vi "Get Property.vi"(0 "Session Handle in":T1, 5 "resources":string, 7 "property":refnum<k21>, 11 "error in (no error)":errorcluster) -> (4 "Session Handle out":T1, 10 "property value":bool, 15 "error out":errorcluster)   [LabVIEW 2015, in "SLSC Switch.lvlib" / "SLSC Session.lvclass"]
uses:
  SLSC Session.lvclass
  Typedefs/Session Handle.ctl
  SLSC Session.lvclass/SLSC Session.ctl
  <vilib>/SLSC/Get Generic Property (Bool).vi
  <vilib>/SLSC/SLSC.lvlib
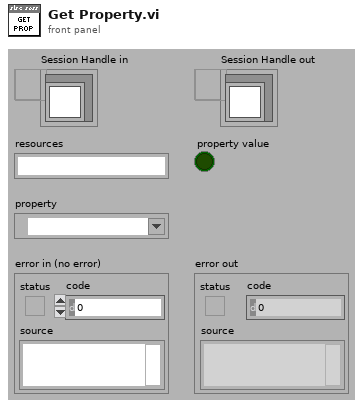
[diagram p1: front panel]
types:
  T1 = typedef "SLSC Switch.lvlib/SLSC Session.lvclass/Session Handle.ctl" = refnum<data-value>
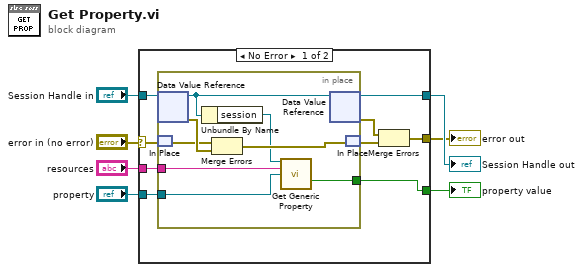
[diagram p0: block diagram]
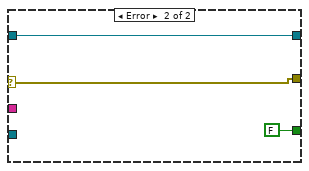
[diagram p2: hidden frame]
diagram:
  n1 = case shown="No Error" "error in (no error)" {
    selector: "error in (no error)" -> [w11 w26]
    tunnel: "Session Handle in" -> [w16 w27]
    tunnel: [w15 w27] -> w6
    tunnel: [w12 w26] -> w5
    tunnel: "property" -> [w10 _]
    tunnel: [w9 FALSE ("property value")] -> w2
    tunnel: "resources" -> [w8 _]
    frame No Error {
      n2 = in-place {
        in-place-border: w10 -> [w19]
        in-place-border: [w18] -> w9
        in-place-border: w8 -> [w17]
        n3 = in-place-dvr #1(w16) -> (w21:refnum<class "SLSC Session.lvclass">, w23:errorcluster)
        n4 = in-place-match #2(w11) -> (w22:errorcluster)
        n5 = Unbundle By Name(w21) -> ("session"=w20:refnum<k21>)
        n6 = Merge Errors(w22, w23) -> (w24:errorcluster)
        n7 = call-poly <vilib>:"Get Generic Property.vi"("session in"=w20, "resources"=w17, "property"=w19) -> ("property value"=w18:bool)  [unwired: 10 in, 2 out]
        n8 = in-place-dvr #1(w21) -> (w15:T1, w13:errorcluster)
        n9 = in-place-match #2(w24) -> (w14:errorcluster)
      }
      n10 = Merge Errors(w13, w14) -> (w12:errorcluster)
    }
    frame Error {
    }
  }
  "Session Handle out" <- w6
  "error out" <- w5
  "property value" <- w2
